vi "Media si dispersia Metoda 2.vi"() -> ()   [LabVIEW 2011]
panel:
  out "Numeric":dbl=4.0
  in  "Baza":dbl(slide)=4.0 scale=0.0..10.0
  out "Valoarea instantanee":dbl
  in  "stop":bool
  out "Suma valorilor":dbl
  out "Numarul de valori":dbl
  out "Dispersia":dbl
  out "Media":dbl
  out "Grafic":dbl(graph) caption="Valoarea instantanee"
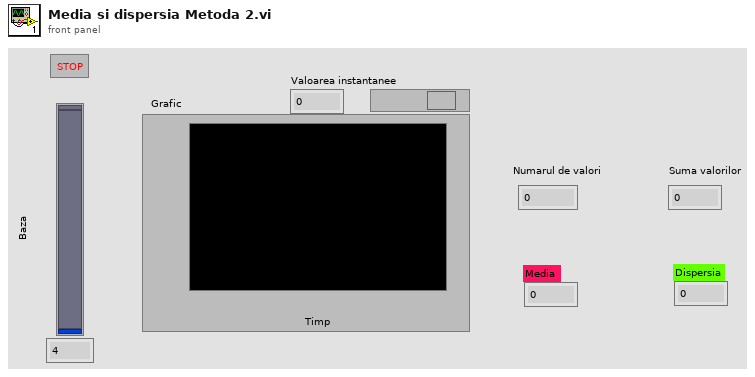
[diagram p1: front panel]
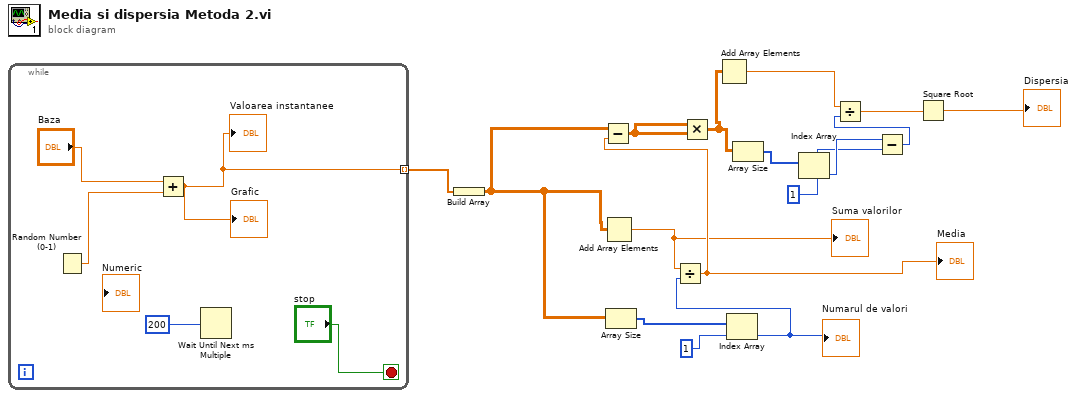
[diagram p0: block diagram]
diagram:
  w3 = 1
  n1 = while {
    tunnel: [w18] -> w8 mode=indexing
    stop <- "stop" stop-if-true
    n2 = Random Number (0-1)() -> (number: 0 to 1=w20:dbl)
    n3 = Add(x="Baza", y=w20) -> (x+y=w18:dbl)
    "Grafic" <- w18
    "Valoarea instantanee" <- w18
    n4 = Wait Until Next ms Multiple(millisecond multiple=200) -> ()  [unwired: 1 out]
  }
  n5 = Build Array "Build Array"(w8) -> (w11:dbl[][])
  n6 = Add Array Elements(numeric array=w11) -> (sum=w7:dbl)
  "Suma valorilor" <- w7
  n7 = Array Size(array=w11) -> (size(s)=w2:i32[])
  n8 = Index Array "Index Array"(array=w2, index=1) -> (element=w1:i32)
  "Numarul de valori" <- w1
  n9 = Divide(x=w7, y=w1) -> (x/y=w9:dbl)
  "Media" <- w9
  n10 = Subtract(x=w11, y=w9) -> (x-y=w16:dbl[][])
  n11 = Multiply(x=w16, y=w16) -> (x*y=w6:dbl[][])
  n12 = Add Array Elements(numeric array=w6) -> (sum=w12:dbl)
  n13 = Array Size(array=w6) -> (size(s)=w4:i32[])
  n14 = Index Array "Index Array"(array=w4, index=w3) -> (element=w5:i32)
  n15 = Subtract(x=w5, y=w3) -> (x-y=w15:i32)
  n16 = Divide(x=w12, y=w15) -> (x/y=w14:dbl)
  n17 = Square Root(x=w14) -> (sqrt(x)=→"Dispersia":dbl)
